vi "Dialog_NoSensor.vi"() -> (5 "OK":bool, 6 "Cancel":bool)   [LabVIEW 2011]
panel:
  out "time":string
  in  "Abort":bool
  in  "stop":bool
  # "Connection lost,\n no sensor connected\nor sensor is not supported\nby PM100 / PM200 device"
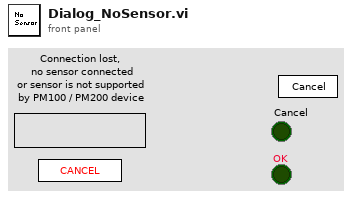
[diagram p1: front panel]
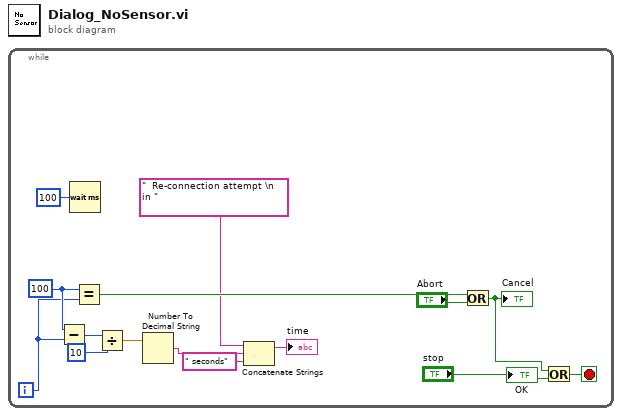
[diagram p0: block diagram]
diagram:
  n1 = while {
    i -> [w8]
    stop <- w14 stop-if-true
    w9 = 100 ("x")
    n2 = Subtract(x=w9, y=w8) -> (x-y=w7:i32)
    n3 = Wait (ms)(milliseconds to wait=u32 100) -> ()  [unwired: 1 out]
    n4 = Equal?(x=w9, y=w8) -> (x = y?=w10:bool)
    n5 = Divide(x=w7, y=10) -> (x/y=w5:dbl)
    n6 = Number To Decimal String(number=w5) -> (decimal integer string=w3:string)  [unwired: 1 in]
    n7 = Concatenate Strings("  Re-connection attempt \n         in " ("string"), w3, " seconds" ("string")) -> (→"time":string)
    n8 = Or(x=w10, y="Abort") -> (x .or. y?=w12:bool)
    "Cancel" <- w12
    n9 = Or(x=w12, y="stop") -> (x .or. y?=w14:bool)
    "OK" <- "stop"
  }
